vi "random_U32.vi"(1 "seed":u32 format="%.0x") -> (0 "random":u32 format="%.0x")   [LabVIEW 2019, in "WebSocket Server Toolkit.lvlib"]
uses:
  WebSocket Server Toolkit.lvlib
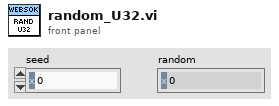
[diagram p1: front panel]
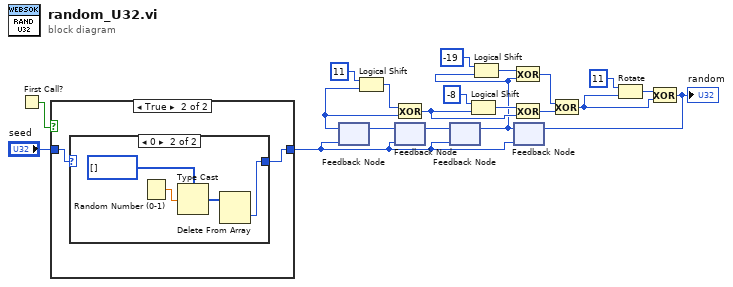
[diagram p0: block diagram]
diagram:
  n1 = First Call?() -> (First Call?: T/F=w9:bool)
  n2 = case shown="True" w9 {
    tunnel: "seed" -> [w21 w23]
    tunnel: [w21 w22] -> w1
    frame False {
    }
    frame True {
      n3 = case shown="0" w23 {
        selector: w23 -> [w24 _]
        tunnel: [w24 w25] -> w22
        frame Default {
        }
        frame 0 {
          n4 = Random Number (0-1)() -> (number: 0 to 1=w27:dbl)
          n5 = Type Cast(type=u32[] [], x=w27) -> (*(type *) &x=w26:u32[])
          n6 = Delete From Array(array=w26) -> (deleted portion=w25:u32)  [unwired: 2 in, 1 out]
        }
      }
    }
  }
  n7 = feedback #1(w1) -> (w3:u32)
  n8 = Logical Shift(y=i16 11, x=w3) -> (x << y=w19:u32)
  n9 = Exclusive Or(1:w3, 2:w19) -> (0:w14:u32)
  n10 = feedback #2(w1) -> (w18:u32)
  n11 = feedback-in #1(w18) -> ()
  n12 = feedback #3(w1) -> (w17:u32)
  n13 = feedback-in #2(w17) -> ()
  n14 = Logical Shift(y=i16 -8, x=w14) -> (x << y=w15:u32)
  n15 = Exclusive Or(1:w14, 2:w15) -> (0:w10:u32)
  n16 = feedback #4(w1) -> (w4:u32)
  n17 = feedback-in #3(w4) -> ()
  n18 = Logical Shift(y=i16 -19, x=w4) -> (x << y=w12:u32)
  n19 = Exclusive Or(1:w4, 2:w12) -> (0:w11:u32)
  n20 = Exclusive Or(1:w10, 2:w11) -> (0:w6:u32)
  n21 = Rotate(1:w6, 2:i16 11 ("y")) -> (0:w7:u32)
  n22 = Exclusive Or(1:w6, 2:w7) -> (0:w5:u32)
  "random" <- w5
  n23 = feedback-in #4(w5) -> ()
